vi "Experiment 24.vi"() -> ()   [LabVIEW 2026]
doc: "Experiment 24\nThis experiment (24) is like experiment 23 but uses 11 loops instead of 10."
uses:
  <vilib>/AdvancedString/1D String Array to Delimited String (string).vi
  <vilib>/Analysis/baseanly.llb/Mean (DBL).vi
  <vilib>/Analysis/NI_AALBase.lvlib
panel:
  out "No. Of Iterations Executed - Loop 11":i32
  out "Output - Loop 11":dbl[](array[numeric]) format="%.3f"
  out "No. Of Iterations As Block Of Text (easy to copy into Excel)":string
  out "No. Of Iterations Executed - Loop 10":i32
  out "Output - Loop 10":dbl[](array[numeric]) format="%.3f"
  out "No. Of Iterations Executed - Loop 9":i32
  out "Output - Loop 9":dbl[](array[numeric]) format="%.3f"
  out "No. Of Iterations Executed - Loop 8":i32
  out "Output - Loop 8":dbl[](array[numeric]) format="%.3f"
  out "No. Of Iterations Executed - Loop 7":i32
  out "Output - Loop 7":dbl[](array[numeric]) format="%.3f"
  out "No. Of Iterations Executed - Loop 6":i32
  out "Output - Loop 6":dbl[](array[numeric]) format="%.3f"
  out "No. Of Iterations Executed - Loop 5":i32
  out "Output - Loop 5":dbl[](array[numeric]) format="%.3f"
  out "No. Of Iterations Executed - Loop 4":i32
  out "Output - Loop 4":dbl[](array[numeric]) format="%.3f"
  out "No. Of Iterations Executed - Loop 3":i32
  out "Output - Loop 3":dbl[](array[numeric]) format="%.3f"
  out "Avg. No. Of Iterations Executed - All Loops":dbl format="%.1f"
  out "No. Of Iterations Executed - Loop 2":i32
  out "Output - Loop 2":dbl[](array[numeric]) format="%.3f"
  out "No. Of Iterations Executed - Loop 1":i32
  out "Output - Loop 1":dbl[](array[numeric]) format="%.3f"
  out "Stop VI?":bool
  # "Experiment 24"
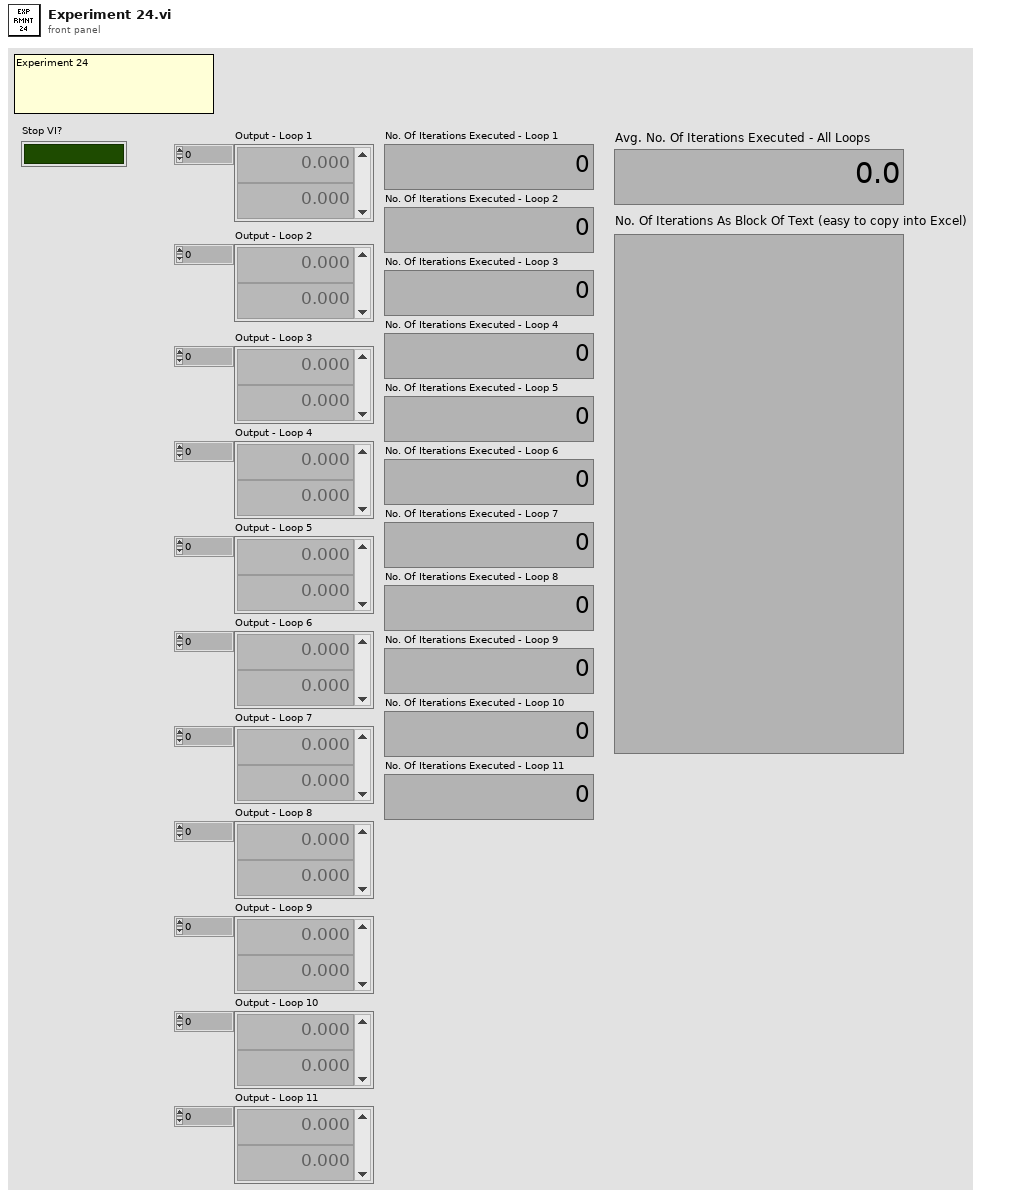
[diagram p1: front panel]
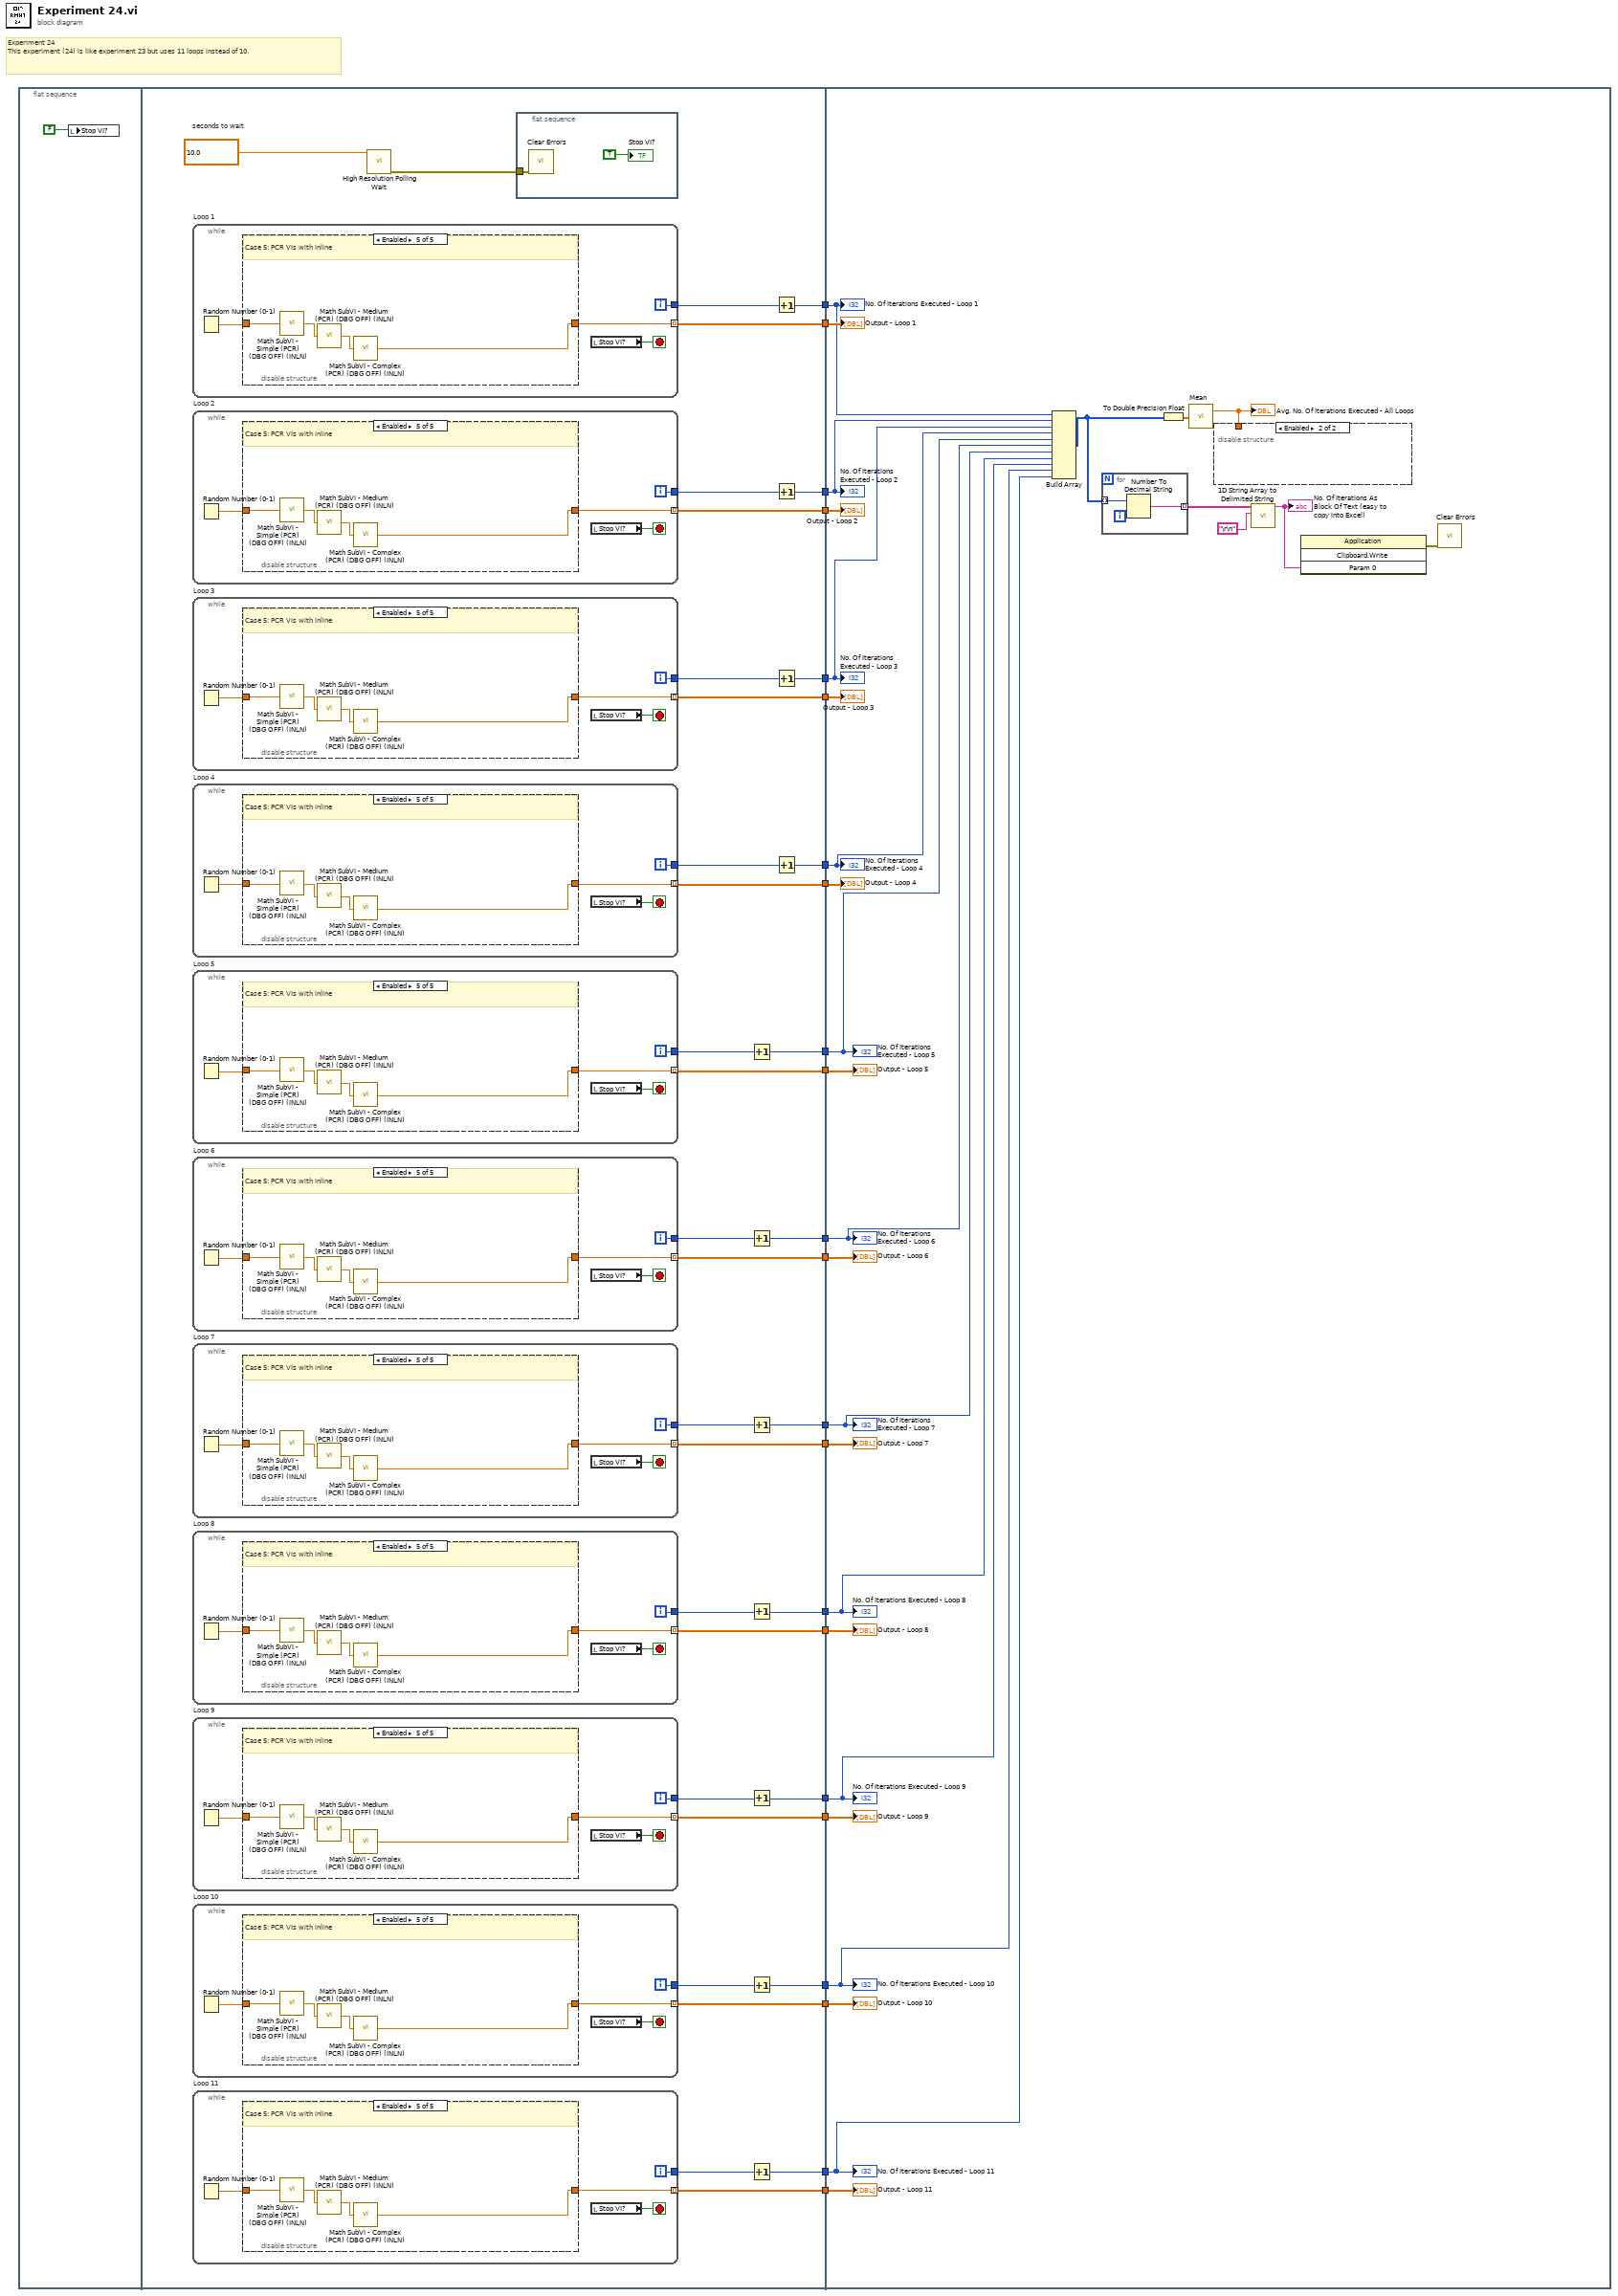
[diagram p0: block diagram]
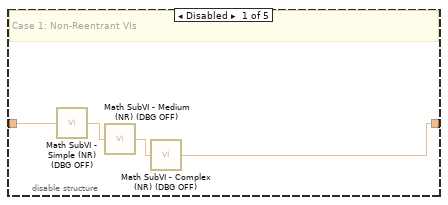
[diagram p2: hidden frame]
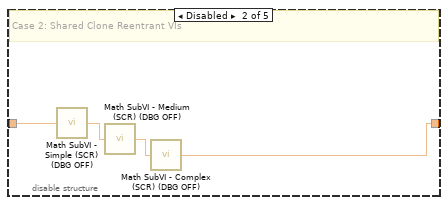
[diagram p3: hidden frame]
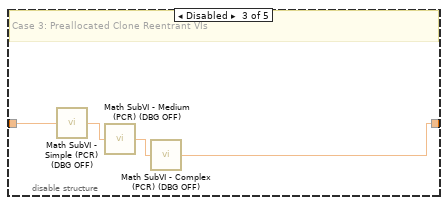
[diagram p4: hidden frame]
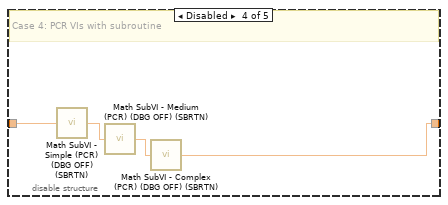
[diagram p5: hidden frame]
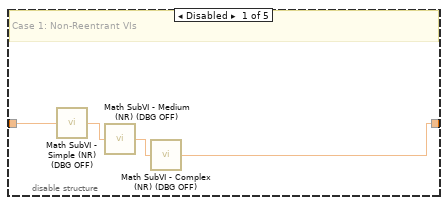
[diagram p6: hidden frame]
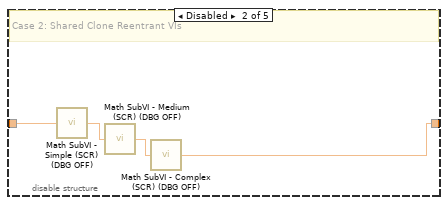
[diagram p7: hidden frame]
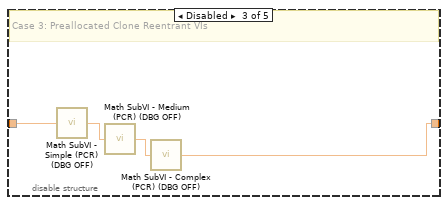
[diagram p8: hidden frame]
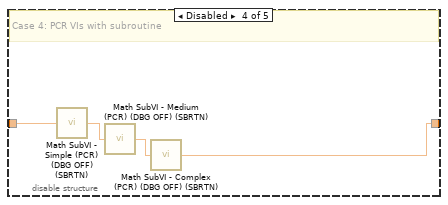
[diagram p9: hidden frame]
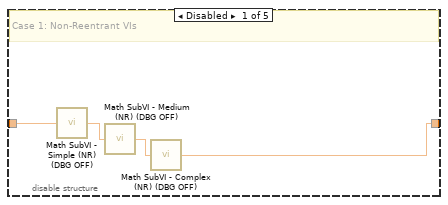
[diagram p10: hidden frame]
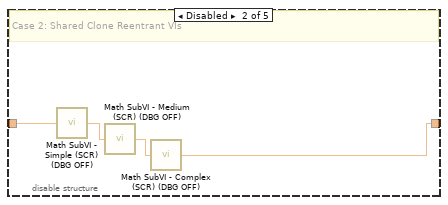
[diagram p11: hidden frame]
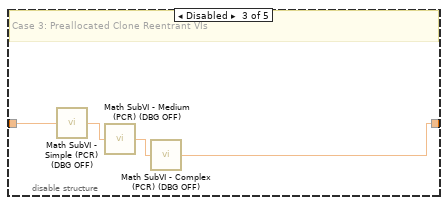
[diagram p12: hidden frame]
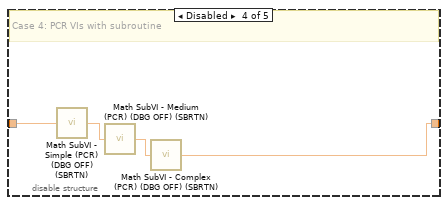
[diagram p13: hidden frame]
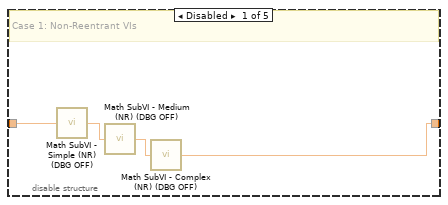
[diagram p14: hidden frame]
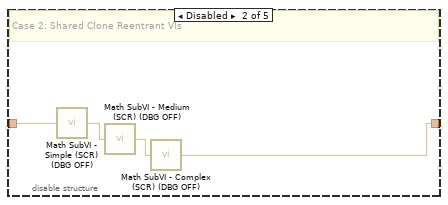
[diagram p15: hidden frame]
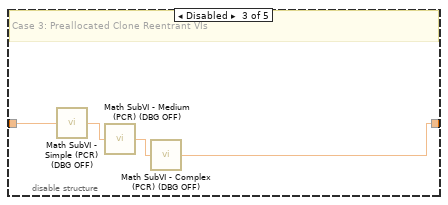
[diagram p16: hidden frame]
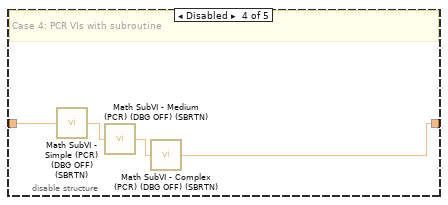
[diagram p17: hidden frame]
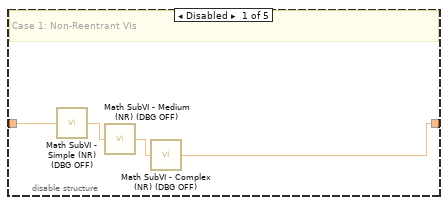
[diagram p18: hidden frame]
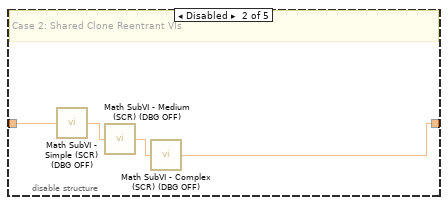
[diagram p19: hidden frame]
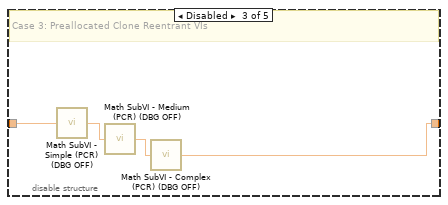
[diagram p20: hidden frame]
diagram:
  # "Experiment 24\nThis experiment (24) is like experiment 23 but uses 11 loops instead of 10."
  n1 = flat-sequence {
    tunnel: [w56] -> w22
    tunnel: [w54] -> w21
    tunnel: [w53] -> w20
    tunnel: [w44] -> w19
    tunnel: [w52] -> w18
    tunnel: [w42] -> w17
    tunnel: [w40] -> w16
    tunnel: [w51] -> w15
    tunnel: [w38] -> w14
    tunnel: [w50] -> w13
    tunnel: [w36] -> w12
    tunnel: [w45] -> w11
    tunnel: [w34] -> w10
    tunnel: [w46] -> w9
    tunnel: [w32] -> w8
    tunnel: [w47] -> w7
    tunnel: [w30] -> w6
    tunnel: [w48] -> w5
    tunnel: [w27] -> w4
    tunnel: [w49] -> w3
    tunnel: [w26] -> w2
    tunnel: [w24] -> w1
    tunnel: w22 -> [w353]
    tunnel: w21 -> [w351]
    tunnel: w20 -> [w350]
    tunnel: w19 -> [w352]
    tunnel: w18 -> [w346]
    tunnel: w17 -> [w348]
    tunnel: w16 -> [w347]
    tunnel: w15 -> [w345]
    tunnel: w14 -> [w343]
    tunnel: w13 -> [w337]
    tunnel: w12 -> [w342]
    tunnel: w11 -> [w336]
    tunnel: w10 -> [w341]
    tunnel: w9 -> [w335]
    tunnel: w8 -> [w340]
    tunnel: w7 -> [w334]
    tunnel: w6 -> [w339]
    tunnel: w5 -> [w333]
    tunnel: w4 -> [w338]
    tunnel: w3 -> [w332]
    tunnel: w2 -> [w326]
    tunnel: w1 -> [w325]
    frame #0 {
      n2 = local write "Stop VI?"(FALSE) -> ()
    }
    frame #1 {
      w58 = 10.0  # seconds to wait
      n3 = while "Loop 1" {
        tunnel: [w300] -> w56 mode=indexing
        tunnel: [w301] -> w55
        i -> [w301]
        stop <- w302 stop-if-true
        n4 = Random Number (0-1)() -> (number: 0 to 1=w299:dbl)
        n5 = disable-structure shown="Enabled" {
          disable-tunnel: w299 -> [w306 w310 w314 w318 w322]
          disable-tunnel: [w305 w309 w313 w317 w321] -> w300
          frame Disabled {
            # "Case 1: Non-Reentrant VIs"
            n6 = call "Math SubVI - Simple (NR) (DBG OFF).vi"("Input"=w306) -> ("Output"=w303:dbl)
            n7 = call "Math SubVI - Medium (NR) (DBG OFF).vi"("Input"=w303) -> ("Output"=w304:dbl)
            n8 = call "Math SubVI - Complex (NR) (DBG OFF).vi"("Input"=w304) -> ("Output"=w305:dbl)
          }
          frame Disabled {
            # "Case 2: Shared Clone Reentrant VIs"
            n9 = call "Math SubVI - Simple (SCR) (DBG OFF).vi"("Input"=w310) -> ("Output"=w307:dbl)
            n10 = call "Math SubVI - Medium (SCR) (DBG OFF).vi"("Input"=w307) -> ("Output"=w308:dbl)
            n11 = call "Math SubVI - Complex (SCR) (DBG OFF).vi"("Input"=w308) -> ("Output"=w309:dbl)
          }
          frame Disabled {
            # "Case 3: Preallocated Clone Reentrant VIs"
            n12 = call "Math SubVI - Simple (PCR) (DBG OFF).vi"("Input"=w314) -> ("Output"=w311:dbl)
            n13 = call "Math SubVI - Medium (PCR) (DBG OFF).vi"("Input"=w311) -> ("Output"=w312:dbl)
            n14 = call "Math SubVI - Complex (PCR) (DBG OFF).vi"("Input"=w312) -> ("Output"=w313:dbl)
          }
          frame Disabled {
            # "Case 4: PCR VIs with subroutine"
            n15 = call "Math SubVI - Simple (PCR) (DBG OFF) (SBRTN).vi"("Input"=w318) -> ("Output"=w315:dbl)
            n16 = call "Math SubVI - Medium (PCR) (DBG OFF) (SBRTN).vi"("Input"=w315) -> ("Output"=w316:dbl)
            n17 = call "Math SubVI - Complex (PCR) (DBG OFF) (SBRTN).vi"("Input"=w316) -> ("Output"=w317:dbl)
          }
          frame Enabled {
            # "Case 5: PCR VIs with inline"
            n18 = call "Math SubVI - Simple (PCR) (DBG OFF) (INLN).vi"("Input"=w322) -> ("Output"=w319:dbl)
            n19 = call "Math SubVI - Medium (PCR) (DBG OFF) (INLN).vi"("Input"=w319) -> ("Output"=w320:dbl)
            n20 = call "Math SubVI - Complex (PCR) (DBG OFF) (INLN).vi"("Input"=w320) -> ("Output"=w321:dbl)
          }
        }
        n21 = local read "Stop VI?"() -> (w302:bool)
      }
      n22 = while "Loop 2" {
        tunnel: [w276] -> w44 mode=indexing
        tunnel: [w277] -> w43
        i -> [w277]
        stop <- w278 stop-if-true
        n23 = Random Number (0-1)() -> (number: 0 to 1=w275:dbl)
        n24 = disable-structure shown="Enabled" {
          disable-tunnel: w275 -> [w282 w286 w290 w294 w298]
          disable-tunnel: [w281 w285 w289 w293 w297] -> w276
          frame Disabled {
            # "Case 1: Non-Reentrant VIs"
            n25 = call "Math SubVI - Simple (NR) (DBG OFF).vi"("Input"=w282) -> ("Output"=w279:dbl)
            n26 = call "Math SubVI - Medium (NR) (DBG OFF).vi"("Input"=w279) -> ("Output"=w280:dbl)
            n27 = call "Math SubVI - Complex (NR) (DBG OFF).vi"("Input"=w280) -> ("Output"=w281:dbl)
          }
          frame Disabled {
            # "Case 2: Shared Clone Reentrant VIs"
            n28 = call "Math SubVI - Simple (SCR) (DBG OFF).vi"("Input"=w286) -> ("Output"=w283:dbl)
            n29 = call "Math SubVI - Medium (SCR) (DBG OFF).vi"("Input"=w283) -> ("Output"=w284:dbl)
            n30 = call "Math SubVI - Complex (SCR) (DBG OFF).vi"("Input"=w284) -> ("Output"=w285:dbl)
          }
          frame Disabled {
            # "Case 3: Preallocated Clone Reentrant VIs"
            n31 = call "Math SubVI - Simple (PCR) (DBG OFF).vi"("Input"=w290) -> ("Output"=w287:dbl)
            n32 = call "Math SubVI - Medium (PCR) (DBG OFF).vi"("Input"=w287) -> ("Output"=w288:dbl)
            n33 = call "Math SubVI - Complex (PCR) (DBG OFF).vi"("Input"=w288) -> ("Output"=w289:dbl)
          }
          frame Disabled {
            # "Case 4: PCR VIs with subroutine"
            n34 = call "Math SubVI - Simple (PCR) (DBG OFF) (SBRTN).vi"("Input"=w294) -> ("Output"=w291:dbl)
            n35 = call "Math SubVI - Medium (PCR) (DBG OFF) (SBRTN).vi"("Input"=w291) -> ("Output"=w292:dbl)
            n36 = call "Math SubVI - Complex (PCR) (DBG OFF) (SBRTN).vi"("Input"=w292) -> ("Output"=w293:dbl)
          }
          frame Enabled {
            # "Case 5: PCR VIs with inline"
            n37 = call "Math SubVI - Simple (PCR) (DBG OFF) (INLN).vi"("Input"=w298) -> ("Output"=w295:dbl)
            n38 = call "Math SubVI - Medium (PCR) (DBG OFF) (INLN).vi"("Input"=w295) -> ("Output"=w296:dbl)
            n39 = call "Math SubVI - Complex (PCR) (DBG OFF) (INLN).vi"("Input"=w296) -> ("Output"=w297:dbl)
          }
        }
        n40 = local read "Stop VI?"() -> (w278:bool)
      }
      n41 = while "Loop 3" {
        tunnel: [w252] -> w42 mode=indexing
        tunnel: [w253] -> w41
        i -> [w253]
        stop <- w254 stop-if-true
        n42 = Random Number (0-1)() -> (number: 0 to 1=w251:dbl)
        n43 = disable-structure shown="Enabled" {
          disable-tunnel: w251 -> [w258 w262 w266 w270 w274]
          disable-tunnel: [w257 w261 w265 w269 w273] -> w252
          frame Disabled {
            # "Case 1: Non-Reentrant VIs"
            n44 = call "Math SubVI - Simple (NR) (DBG OFF).vi"("Input"=w258) -> ("Output"=w255:dbl)
            n45 = call "Math SubVI - Medium (NR) (DBG OFF).vi"("Input"=w255) -> ("Output"=w256:dbl)
            n46 = call "Math SubVI - Complex (NR) (DBG OFF).vi"("Input"=w256) -> ("Output"=w257:dbl)
          }
          frame Disabled {
            # "Case 2: Shared Clone Reentrant VIs"
            n47 = call "Math SubVI - Simple (SCR) (DBG OFF).vi"("Input"=w262) -> ("Output"=w259:dbl)
            n48 = call "Math SubVI - Medium (SCR) (DBG OFF).vi"("Input"=w259) -> ("Output"=w260:dbl)
            n49 = call "Math SubVI - Complex (SCR) (DBG OFF).vi"("Input"=w260) -> ("Output"=w261:dbl)
          }
          frame Disabled {
            # "Case 3: Preallocated Clone Reentrant VIs"
            n50 = call "Math SubVI - Simple (PCR) (DBG OFF).vi"("Input"=w266) -> ("Output"=w263:dbl)
            n51 = call "Math SubVI - Medium (PCR) (DBG OFF).vi"("Input"=w263) -> ("Output"=w264:dbl)
            n52 = call "Math SubVI - Complex (PCR) (DBG OFF).vi"("Input"=w264) -> ("Output"=w265:dbl)
          }
          frame Disabled {
            # "Case 4: PCR VIs with subroutine"
            n53 = call "Math SubVI - Simple (PCR) (DBG OFF) (SBRTN).vi"("Input"=w270) -> ("Output"=w267:dbl)
            n54 = call "Math SubVI - Medium (PCR) (DBG OFF) (SBRTN).vi"("Input"=w267) -> ("Output"=w268:dbl)
            n55 = call "Math SubVI - Complex (PCR) (DBG OFF) (SBRTN).vi"("Input"=w268) -> ("Output"=w269:dbl)
          }
          frame Enabled {
            # "Case 5: PCR VIs with inline"
            n56 = call "Math SubVI - Simple (PCR) (DBG OFF) (INLN).vi"("Input"=w274) -> ("Output"=w271:dbl)
            n57 = call "Math SubVI - Medium (PCR) (DBG OFF) (INLN).vi"("Input"=w271) -> ("Output"=w272:dbl)
            n58 = call "Math SubVI - Complex (PCR) (DBG OFF) (INLN).vi"("Input"=w272) -> ("Output"=w273:dbl)
          }
        }
        n59 = local read "Stop VI?"() -> (w254:bool)
      }
      n60 = while "Loop 4" {
        tunnel: [w228] -> w40 mode=indexing
        tunnel: [w229] -> w39
        i -> [w229]
        stop <- w230 stop-if-true
        n61 = Random Number (0-1)() -> (number: 0 to 1=w227:dbl)
        n62 = disable-structure shown="Enabled" {
          disable-tunnel: w227 -> [w234 w238 w242 w246 w250]
          disable-tunnel: [w233 w237 w241 w245 w249] -> w228
          frame Disabled {
            # "Case 1: Non-Reentrant VIs"
            n63 = call "Math SubVI - Simple (NR) (DBG OFF).vi"("Input"=w234) -> ("Output"=w231:dbl)
            n64 = call "Math SubVI - Medium (NR) (DBG OFF).vi"("Input"=w231) -> ("Output"=w232:dbl)
            n65 = call "Math SubVI - Complex (NR) (DBG OFF).vi"("Input"=w232) -> ("Output"=w233:dbl)
          }
          frame Disabled {
            # "Case 2: Shared Clone Reentrant VIs"
            n66 = call "Math SubVI - Simple (SCR) (DBG OFF).vi"("Input"=w238) -> ("Output"=w235:dbl)
            n67 = call "Math SubVI - Medium (SCR) (DBG OFF).vi"("Input"=w235) -> ("Output"=w236:dbl)
            n68 = call "Math SubVI - Complex (SCR) (DBG OFF).vi"("Input"=w236) -> ("Output"=w237:dbl)
          }
          frame Disabled {
            # "Case 3: Preallocated Clone Reentrant VIs"
            n69 = call "Math SubVI - Simple (PCR) (DBG OFF).vi"("Input"=w242) -> ("Output"=w239:dbl)
            n70 = call "Math SubVI - Medium (PCR) (DBG OFF).vi"("Input"=w239) -> ("Output"=w240:dbl)
            n71 = call "Math SubVI - Complex (PCR) (DBG OFF).vi"("Input"=w240) -> ("Output"=w241:dbl)
          }
          frame Disabled {
            # "Case 4: PCR VIs with subroutine"
            n72 = call "Math SubVI - Simple (PCR) (DBG OFF) (SBRTN).vi"("Input"=w246) -> ("Output"=w243:dbl)
            n73 = call "Math SubVI - Medium (PCR) (DBG OFF) (SBRTN).vi"("Input"=w243) -> ("Output"=w244:dbl)
            n74 = call "Math SubVI - Complex (PCR) (DBG OFF) (SBRTN).vi"("Input"=w244) -> ("Output"=w245:dbl)
          }
          frame Enabled {
            # "Case 5: PCR VIs with inline"
            n75 = call "Math SubVI - Simple (PCR) (DBG OFF) (INLN).vi"("Input"=w250) -> ("Output"=w247:dbl)
            n76 = call "Math SubVI - Medium (PCR) (DBG OFF) (INLN).vi"("Input"=w247) -> ("Output"=w248:dbl)
            n77 = call "Math SubVI - Complex (PCR) (DBG OFF) (INLN).vi"("Input"=w248) -> ("Output"=w249:dbl)
          }
        }
        n78 = local read "Stop VI?"() -> (w230:bool)
      }
      n79 = while "Loop 5" {
        tunnel: [w204] -> w38 mode=indexing
        tunnel: [w205] -> w37
        i -> [w205]
        stop <- w206 stop-if-true
        n80 = Random Number (0-1)() -> (number: 0 to 1=w203:dbl)
        n81 = disable-structure shown="Enabled" {
          disable-tunnel: w203 -> [w210 w214 w218 w222 w226]
          disable-tunnel: [w209 w213 w217 w221 w225] -> w204
          frame Disabled {
            # "Case 1: Non-Reentrant VIs"
            n82 = call "Math SubVI - Simple (NR) (DBG OFF).vi"("Input"=w210) -> ("Output"=w207:dbl)
            n83 = call "Math SubVI - Medium (NR) (DBG OFF).vi"("Input"=w207) -> ("Output"=w208:dbl)
            n84 = call "Math SubVI - Complex (NR) (DBG OFF).vi"("Input"=w208) -> ("Output"=w209:dbl)
          }
          frame Disabled {
            # "Case 2: Shared Clone Reentrant VIs"
            n85 = call "Math SubVI - Simple (SCR) (DBG OFF).vi"("Input"=w214) -> ("Output"=w211:dbl)
            n86 = call "Math SubVI - Medium (SCR) (DBG OFF).vi"("Input"=w211) -> ("Output"=w212:dbl)
            n87 = call "Math SubVI - Complex (SCR) (DBG OFF).vi"("Input"=w212) -> ("Output"=w213:dbl)
          }
          frame Disabled {
            # "Case 3: Preallocated Clone Reentrant VIs"
            n88 = call "Math SubVI - Simple (PCR) (DBG OFF).vi"("Input"=w218) -> ("Output"=w215:dbl)
            n89 = call "Math SubVI - Medium (PCR) (DBG OFF).vi"("Input"=w215) -> ("Output"=w216:dbl)
            n90 = call "Math SubVI - Complex (PCR) (DBG OFF).vi"("Input"=w216) -> ("Output"=w217:dbl)
          }
          frame Disabled {
            # "Case 4: PCR VIs with subroutine"
            n91 = call "Math SubVI - Simple (PCR) (DBG OFF) (SBRTN).vi"("Input"=w222) -> ("Output"=w219:dbl)
            n92 = call "Math SubVI - Medium (PCR) (DBG OFF) (SBRTN).vi"("Input"=w219) -> ("Output"=w220:dbl)
            n93 = call "Math SubVI - Complex (PCR) (DBG OFF) (SBRTN).vi"("Input"=w220) -> ("Output"=w221:dbl)
          }
          frame Enabled {
            # "Case 5: PCR VIs with inline"
            n94 = call "Math SubVI - Simple (PCR) (DBG OFF) (INLN).vi"("Input"=w226) -> ("Output"=w223:dbl)
            n95 = call "Math SubVI - Medium (PCR) (DBG OFF) (INLN).vi"("Input"=w223) -> ("Output"=w224:dbl)
            n96 = call "Math SubVI - Complex (PCR) (DBG OFF) (INLN).vi"("Input"=w224) -> ("Output"=w225:dbl)
          }
        }
        n97 = local read "Stop VI?"() -> (w206:bool)
      }
      n98 = while "Loop 6" {
        tunnel: [w180] -> w36 mode=indexing
        tunnel: [w181] -> w35
        i -> [w181]
        stop <- w182 stop-if-true
        n99 = Random Number (0-1)() -> (number: 0 to 1=w179:dbl)
        n100 = disable-structure shown="Enabled" {
          disable-tunnel: w179 -> [w186 w190 w194 w198 w202]
          disable-tunnel: [w185 w189 w193 w197 w201] -> w180
          frame Disabled {
            # "Case 1: Non-Reentrant VIs"
            n101 = call "Math SubVI - Simple (NR) (DBG OFF).vi"("Input"=w186) -> ("Output"=w183:dbl)
            n102 = call "Math SubVI - Medium (NR) (DBG OFF).vi"("Input"=w183) -> ("Output"=w184:dbl)
            n103 = call "Math SubVI - Complex (NR) (DBG OFF).vi"("Input"=w184) -> ("Output"=w185:dbl)
          }
          frame Disabled {
            # "Case 2: Shared Clone Reentrant VIs"
            n104 = call "Math SubVI - Simple (SCR) (DBG OFF).vi"("Input"=w190) -> ("Output"=w187:dbl)
            n105 = call "Math SubVI - Medium (SCR) (DBG OFF).vi"("Input"=w187) -> ("Output"=w188:dbl)
            n106 = call "Math SubVI - Complex (SCR) (DBG OFF).vi"("Input"=w188) -> ("Output"=w189:dbl)
          }
          frame Disabled {
            # "Case 3: Preallocated Clone Reentrant VIs"
            n107 = call "Math SubVI - Simple (PCR) (DBG OFF).vi"("Input"=w194) -> ("Output"=w191:dbl)
            n108 = call "Math SubVI - Medium (PCR) (DBG OFF).vi"("Input"=w191) -> ("Output"=w192:dbl)
            n109 = call "Math SubVI - Complex (PCR) (DBG OFF).vi"("Input"=w192) -> ("Output"=w193:dbl)
          }
          frame Disabled {
            # "Case 4: PCR VIs with subroutine"
            n110 = call "Math SubVI - Simple (PCR) (DBG OFF) (SBRTN).vi"("Input"=w198) -> ("Output"=w195:dbl)
            n111 = call "Math SubVI - Medium (PCR) (DBG OFF) (SBRTN).vi"("Input"=w195) -> ("Output"=w196:dbl)
            n112 = call "Math SubVI - Complex (PCR) (DBG OFF) (SBRTN).vi"("Input"=w196) -> ("Output"=w197:dbl)
          }
          frame Enabled {
            # "Case 5: PCR VIs with inline"
            n113 = call "Math SubVI - Simple (PCR) (DBG OFF) (INLN).vi"("Input"=w202) -> ("Output"=w199:dbl)
            n114 = call "Math SubVI - Medium (PCR) (DBG OFF) (INLN).vi"("Input"=w199) -> ("Output"=w200:dbl)
            n115 = call "Math SubVI - Complex (PCR) (DBG OFF) (INLN).vi"("Input"=w200) -> ("Output"=w201:dbl)
          }
        }
        n116 = local read "Stop VI?"() -> (w182:bool)
      }
      n117 = while "Loop 7" {
        tunnel: [w156] -> w34 mode=indexing
        tunnel: [w157] -> w33
        i -> [w157]
        stop <- w158 stop-if-true
        n118 = Random Number (0-1)() -> (number: 0 to 1=w155:dbl)
        n119 = disable-structure shown="Enabled" {
          disable-tunnel: w155 -> [w162 w166 w170 w174 w178]
          disable-tunnel: [w161 w165 w169 w173 w177] -> w156
          frame Disabled {
            # "Case 1: Non-Reentrant VIs"
            n120 = call "Math SubVI - Simple (NR) (DBG OFF).vi"("Input"=w162) -> ("Output"=w159:dbl)
            n121 = call "Math SubVI - Medium (NR) (DBG OFF).vi"("Input"=w159) -> ("Output"=w160:dbl)
            n122 = call "Math SubVI - Complex (NR) (DBG OFF).vi"("Input"=w160) -> ("Output"=w161:dbl)
          }
          frame Disabled {
            # "Case 2: Shared Clone Reentrant VIs"
            n123 = call "Math SubVI - Simple (SCR) (DBG OFF).vi"("Input"=w166) -> ("Output"=w163:dbl)
            n124 = call "Math SubVI - Medium (SCR) (DBG OFF).vi"("Input"=w163) -> ("Output"=w164:dbl)
            n125 = call "Math SubVI - Complex (SCR) (DBG OFF).vi"("Input"=w164) -> ("Output"=w165:dbl)
          }
          frame Disabled {
            # "Case 3: Preallocated Clone Reentrant VIs"
            n126 = call "Math SubVI - Simple (PCR) (DBG OFF).vi"("Input"=w170) -> ("Output"=w167:dbl)
            n127 = call "Math SubVI - Medium (PCR) (DBG OFF).vi"("Input"=w167) -> ("Output"=w168:dbl)
            n128 = call "Math SubVI - Complex (PCR) (DBG OFF).vi"("Input"=w168) -> ("Output"=w169:dbl)
          }
          frame Disabled {
            # "Case 4: PCR VIs with subroutine"
            n129 = call "Math SubVI - Simple (PCR) (DBG OFF) (SBRTN).vi"("Input"=w174) -> ("Output"=w171:dbl)
            n130 = call "Math SubVI - Medium (PCR) (DBG OFF) (SBRTN).vi"("Input"=w171) -> ("Output"=w172:dbl)
            n131 = call "Math SubVI - Complex (PCR) (DBG OFF) (SBRTN).vi"("Input"=w172) -> ("Output"=w173:dbl)
          }
          frame Enabled {
            # "Case 5: PCR VIs with inline"
            n132 = call "Math SubVI - Simple (PCR) (DBG OFF) (INLN).vi"("Input"=w178) -> ("Output"=w175:dbl)
            n133 = call "Math SubVI - Medium (PCR) (DBG OFF) (INLN).vi"("Input"=w175) -> ("Output"=w176:dbl)
            n134 = call "Math SubVI - Complex (PCR) (DBG OFF) (INLN).vi"("Input"=w176) -> ("Output"=w177:dbl)
          }
        }
        n135 = local read "Stop VI?"() -> (w158:bool)
      }
      n136 = while "Loop 8" {
        tunnel: [w132] -> w32 mode=indexing
        tunnel: [w133] -> w31
        i -> [w133]
        stop <- w134 stop-if-true
        n137 = Random Number (0-1)() -> (number: 0 to 1=w131:dbl)
        n138 = disable-structure shown="Enabled" {
          disable-tunnel: w131 -> [w138 w142 w146 w150 w154]
          disable-tunnel: [w137 w141 w145 w149 w153] -> w132
          frame Disabled {
            # "Case 1: Non-Reentrant VIs"
            n139 = call "Math SubVI - Simple (NR) (DBG OFF).vi"("Input"=w138) -> ("Output"=w135:dbl)
            n140 = call "Math SubVI - Medium (NR) (DBG OFF).vi"("Input"=w135) -> ("Output"=w136:dbl)
            n141 = call "Math SubVI - Complex (NR) (DBG OFF).vi"("Input"=w136) -> ("Output"=w137:dbl)
          }
          frame Disabled {
            # "Case 2: Shared Clone Reentrant VIs"
            n142 = call "Math SubVI - Simple (SCR) (DBG OFF).vi"("Input"=w142) -> ("Output"=w139:dbl)
            n143 = call "Math SubVI - Medium (SCR) (DBG OFF).vi"("Input"=w139) -> ("Output"=w140:dbl)
            n144 = call "Math SubVI - Complex (SCR) (DBG OFF).vi"("Input"=w140) -> ("Output"=w141:dbl)
          }
          frame Disabled {
            # "Case 3: Preallocated Clone Reentrant VIs"
            n145 = call "Math SubVI - Simple (PCR) (DBG OFF).vi"("Input"=w146) -> ("Output"=w143:dbl)
            n146 = call "Math SubVI - Medium (PCR) (DBG OFF).vi"("Input"=w143) -> ("Output"=w144:dbl)
            n147 = call "Math SubVI - Complex (PCR) (DBG OFF).vi"("Input"=w144) -> ("Output"=w145:dbl)
          }
          frame Disabled {
            # "Case 4: PCR VIs with subroutine"
            n148 = call "Math SubVI - Simple (PCR) (DBG OFF) (SBRTN).vi"("Input"=w150) -> ("Output"=w147:dbl)
            n149 = call "Math SubVI - Medium (PCR) (DBG OFF) (SBRTN).vi"("Input"=w147) -> ("Output"=w148:dbl)
            n150 = call "Math SubVI - Complex (PCR) (DBG OFF) (SBRTN).vi"("Input"=w148) -> ("Output"=w149:dbl)
          }
          frame Enabled {
            # "Case 5: PCR VIs with inline"
            n151 = call "Math SubVI - Simple (PCR) (DBG OFF) (INLN).vi"("Input"=w154) -> ("Output"=w151:dbl)
            n152 = call "Math SubVI - Medium (PCR) (DBG OFF) (INLN).vi"("Input"=w151) -> ("Output"=w152:dbl)
            n153 = call "Math SubVI - Complex (PCR) (DBG OFF) (INLN).vi"("Input"=w152) -> ("Output"=w153:dbl)
          }
        }
        n154 = local read "Stop VI?"() -> (w134:bool)
      }
      n155 = while "Loop 9" {
        tunnel: [w108] -> w30 mode=indexing
        tunnel: [w109] -> w29
        i -> [w109]
        stop <- w110 stop-if-true
        n156 = Random Number (0-1)() -> (number: 0 to 1=w107:dbl)
        n157 = disable-structure shown="Enabled" {
          disable-tunnel: w107 -> [w114 w118 w122 w126 w130]
          disable-tunnel: [w113 w117 w121 w125 w129] -> w108
          frame Disabled {
            # "Case 1: Non-Reentrant VIs"
            n158 = call "Math SubVI - Simple (NR) (DBG OFF).vi"("Input"=w114) -> ("Output"=w111:dbl)
            n159 = call "Math SubVI - Medium (NR) (DBG OFF).vi"("Input"=w111) -> ("Output"=w112:dbl)
            n160 = call "Math SubVI - Complex (NR) (DBG OFF).vi"("Input"=w112) -> ("Output"=w113:dbl)
          }
          frame Disabled {
            # "Case 2: Shared Clone Reentrant VIs"
            n161 = call "Math SubVI - Simple (SCR) (DBG OFF).vi"("Input"=w118) -> ("Output"=w115:dbl)
            n162 = call "Math SubVI - Medium (SCR) (DBG OFF).vi"("Input"=w115) -> ("Output"=w116:dbl)
            n163 = call "Math SubVI - Complex (SCR) (DBG OFF).vi"("Input"=w116) -> ("Output"=w117:dbl)
          }
          frame Disabled {
            # "Case 3: Preallocated Clone Reentrant VIs"
            n164 = call "Math SubVI - Simple (PCR) (DBG OFF).vi"("Input"=w122) -> ("Output"=w119:dbl)
            n165 = call "Math SubVI - Medium (PCR) (DBG OFF).vi"("Input"=w119) -> ("Output"=w120:dbl)
            n166 = call "Math SubVI - Complex (PCR) (DBG OFF).vi"("Input"=w120) -> ("Output"=w121:dbl)
          }
          frame Disabled {
            # "Case 4: PCR VIs with subroutine"
            n167 = call "Math SubVI - Simple (PCR) (DBG OFF) (SBRTN).vi"("Input"=w126) -> ("Output"=w123:dbl)
            n168 = call "Math SubVI - Medium (PCR) (DBG OFF) (SBRTN).vi"("Input"=w123) -> ("Output"=w124:dbl)
            n169 = call "Math SubVI - Complex (PCR) (DBG OFF) (SBRTN).vi"("Input"=w124) -> ("Output"=w125:dbl)
          }
          frame Enabled {
            # "Case 5: PCR VIs with inline"
            n170 = call "Math SubVI - Simple (PCR) (DBG OFF) (INLN).vi"("Input"=w130) -> ("Output"=w127:dbl)
            n171 = call "Math SubVI - Medium (PCR) (DBG OFF) (INLN).vi"("Input"=w127) -> ("Output"=w128:dbl)
            n172 = call "Math SubVI - Complex (PCR) (DBG OFF) (INLN).vi"("Input"=w128) -> ("Output"=w129:dbl)
          }
        }
        n173 = local read "Stop VI?"() -> (w110:bool)
      }
      n174 = while "Loop 10" {
        tunnel: [w84] -> w27 mode=indexing
        tunnel: [w85] -> w28
        i -> [w85]
        stop <- w86 stop-if-true
        n175 = Random Number (0-1)() -> (number: 0 to 1=w83:dbl)
        n176 = disable-structure shown="Enabled" {
          disable-tunnel: w83 -> [w90 w94 w98 w102 w106]
          disable-tunnel: [w89 w93 w97 w101 w105] -> w84
          frame Disabled {
            # "Case 1: Non-Reentrant VIs"
            n177 = call "Math SubVI - Simple (NR) (DBG OFF).vi"("Input"=w90) -> ("Output"=w87:dbl)
            n178 = call "Math SubVI - Medium (NR) (DBG OFF).vi"("Input"=w87) -> ("Output"=w88:dbl)
            n179 = call "Math SubVI - Complex (NR) (DBG OFF).vi"("Input"=w88) -> ("Output"=w89:dbl)
          }
          frame Disabled {
            # "Case 2: Shared Clone Reentrant VIs"
            n180 = call "Math SubVI - Simple (SCR) (DBG OFF).vi"("Input"=w94) -> ("Output"=w91:dbl)
            n181 = call "Math SubVI - Medium (SCR) (DBG OFF).vi"("Input"=w91) -> ("Output"=w92:dbl)
            n182 = call "Math SubVI - Complex (SCR) (DBG OFF).vi"("Input"=w92) -> ("Output"=w93:dbl)
          }
          frame Disabled {
            # "Case 3: Preallocated Clone Reentrant VIs"
            n183 = call "Math SubVI - Simple (PCR) (DBG OFF).vi"("Input"=w98) -> ("Output"=w95:dbl)
            n184 = call "Math SubVI - Medium (PCR) (DBG OFF).vi"("Input"=w95) -> ("Output"=w96:dbl)
            n185 = call "Math SubVI - Complex (PCR) (DBG OFF).vi"("Input"=w96) -> ("Output"=w97:dbl)
          }
          frame Disabled {
            # "Case 4: PCR VIs with subroutine"
            n186 = call "Math SubVI - Simple (PCR) (DBG OFF) (SBRTN).vi"("Input"=w102) -> ("Output"=w99:dbl)
            n187 = call "Math SubVI - Medium (PCR) (DBG OFF) (SBRTN).vi"("Input"=w99) -> ("Output"=w100:dbl)
            n188 = call "Math SubVI - Complex (PCR) (DBG OFF) (SBRTN).vi"("Input"=w100) -> ("Output"=w101:dbl)
          }
          frame Enabled {
            # "Case 5: PCR VIs with inline"
            n189 = call "Math SubVI - Simple (PCR) (DBG OFF) (INLN).vi"("Input"=w106) -> ("Output"=w103:dbl)
            n190 = call "Math SubVI - Medium (PCR) (DBG OFF) (INLN).vi"("Input"=w103) -> ("Output"=w104:dbl)
            n191 = call "Math SubVI - Complex (PCR) (DBG OFF) (INLN).vi"("Input"=w104) -> ("Output"=w105:dbl)
          }
        }
        n192 = local read "Stop VI?"() -> (w86:bool)
      }
      n193 = while "Loop 11" {
        tunnel: [w60] -> w26 mode=indexing
        tunnel: [w61] -> w25
        i -> [w61]
        stop <- w62 stop-if-true
        n194 = Random Number (0-1)() -> (number: 0 to 1=w59:dbl)
        n195 = disable-structure shown="Enabled" {
          disable-tunnel: w59 -> [w66 w70 w74 w78 w82]
          disable-tunnel: [w65 w69 w73 w77 w81] -> w60
          frame Disabled {
            # "Case 1: Non-Reentrant VIs"
            n196 = call "Math SubVI - Simple (NR) (DBG OFF).vi"("Input"=w66) -> ("Output"=w63:dbl)
            n197 = call "Math SubVI - Medium (NR) (DBG OFF).vi"("Input"=w63) -> ("Output"=w64:dbl)
            n198 = call "Math SubVI - Complex (NR) (DBG OFF).vi"("Input"=w64) -> ("Output"=w65:dbl)
          }
          frame Disabled {
            # "Case 2: Shared Clone Reentrant VIs"
            n199 = call "Math SubVI - Simple (SCR) (DBG OFF).vi"("Input"=w70) -> ("Output"=w67:dbl)
            n200 = call "Math SubVI - Medium (SCR) (DBG OFF).vi"("Input"=w67) -> ("Output"=w68:dbl)
            n201 = call "Math SubVI - Complex (SCR) (DBG OFF).vi"("Input"=w68) -> ("Output"=w69:dbl)
          }
          frame Disabled {
            # "Case 3: Preallocated Clone Reentrant VIs"
            n202 = call "Math SubVI - Simple (PCR) (DBG OFF).vi"("Input"=w74) -> ("Output"=w71:dbl)
            n203 = call "Math SubVI - Medium (PCR) (DBG OFF).vi"("Input"=w71) -> ("Output"=w72:dbl)
            n204 = call "Math SubVI - Complex (PCR) (DBG OFF).vi"("Input"=w72) -> ("Output"=w73:dbl)
          }
          frame Disabled {
            # "Case 4: PCR VIs with subroutine"
            n205 = call "Math SubVI - Simple (PCR) (DBG OFF) (SBRTN).vi"("Input"=w78) -> ("Output"=w75:dbl)
            n206 = call "Math SubVI - Medium (PCR) (DBG OFF) (SBRTN).vi"("Input"=w75) -> ("Output"=w76:dbl)
            n207 = call "Math SubVI - Complex (PCR) (DBG OFF) (SBRTN).vi"("Input"=w76) -> ("Output"=w77:dbl)
          }
          frame Enabled {
            # "Case 5: PCR VIs with inline"
            n208 = call "Math SubVI - Simple (PCR) (DBG OFF) (INLN).vi"("Input"=w82) -> ("Output"=w79:dbl)
            n209 = call "Math SubVI - Medium (PCR) (DBG OFF) (INLN).vi"("Input"=w79) -> ("Output"=w80:dbl)
            n210 = call "Math SubVI - Complex (PCR) (DBG OFF) (INLN).vi"("Input"=w80) -> ("Output"=w81:dbl)
          }
        }
        n211 = local read "Stop VI?"() -> (w62:bool)
      }
      n212 = call <vilib>:"High Resolution Polling Wait.vi"("seconds to wait"=w58) -> ("error out"=w57:errorcluster)  [unwired: 10 in]
      n213 = flat-sequence {
        tunnel: w57 -> [w323]
        frame #0 {
          n214 = call <vilib>:"Clear Errors.vi"("error in (no error)"=w323) -> ()  [unwired: 5 in, 2 out]
          "Stop VI?" <- TRUE
        }
      }
      n215 = Increment(x=w37) -> (x+1=w50:i32)
      n216 = Increment(x=w35) -> (x+1=w45:i32)
      n217 = Increment(x=w33) -> (x+1=w46:i32)
      n218 = Increment(x=w31) -> (x+1=w47:i32)
      n219 = Increment(x=w29) -> (x+1=w48:i32)
      n220 = Increment(x=w28) -> (x+1=w49:i32)
      n221 = Increment(x=w25) -> (x+1=w24:i32)
      n222 = Increment(x=w55) -> (x+1=w54:i32)
      n223 = Increment(x=w43) -> (x+1=w53:i32)
      n224 = Increment(x=w41) -> (x+1=w52:i32)
      n225 = Increment(x=w39) -> (x+1=w51:i32)
    }
    frame #2 {
      n226 = Build Array(w351, w350, w346, w345, w337, w336, w335, w334, w333, w332, w325) -> (w331:i32[])
      n227 = for {
        tunnel: w331 -> [w357] mode=indexing
        tunnel: [w356] -> w330 mode=indexing
        n228 = Number To Decimal String(number=w357) -> (decimal integer string=w356:string)  [unwired: 1 in]
      }
      n229 = To Double Precision Float(number=w331) -> (double precision float=w344:dbl[])
      n230 = call-poly <vilib>:"Mean.vi"("X"=w344) -> ("mean"=w349:dbl)  [unwired: 1 out]
      "Avg. No. Of Iterations Executed - All Loops" <- w349
      n231 = disable-structure shown="Enabled" {
        disable-tunnel: w349 -> [w355 _]
        frame Disabled {
          n232 = call "Copy Result To Clipboard.vi"("No. Of Decimal Places (6)"=u32 1, "Input"=w355) -> ()
        }
        frame Enabled {
        }
      }
      n233 = call-poly <vilib>:"1D String Array to Delimited String.vi"("delimiter"="\r\n", "string array"=w330) -> ("delimited string"=w327:string)  [unwired: 9 in]
      "No. Of Iterations As Block Of Text (easy to copy into Excel)" <- w327
      n234 = invoke class="Application" method="Clipboard.Write"("Param 0"=w327) -> (error out=w328:errorcluster)  [unwired: 3 in, 3 out]
      n235 = call <vilib>:"Clear Errors.vi"("error in (no error)"=w328) -> ()  [unwired: 5 in, 2 out]
      "No. Of Iterations Executed - Loop 1" <- w351
      "Output - Loop 1" <- w353
      "No. Of Iterations Executed - Loop 2" <- w350
      "Output - Loop 2" <- w352
      "No. Of Iterations Executed - Loop 3" <- w346
      "Output - Loop 3" <- w348
      "No. Of Iterations Executed - Loop 4" <- w345
      "Output - Loop 4" <- w347
      "No. Of Iterations Executed - Loop 5" <- w337
      "Output - Loop 5" <- w343
      "No. Of Iterations Executed - Loop 6" <- w336
      "Output - Loop 6" <- w342
      "No. Of Iterations Executed - Loop 7" <- w335
      "Output - Loop 7" <- w341
      "No. Of Iterations Executed - Loop 8" <- w334
      "Output - Loop 8" <- w340
      "No. Of Iterations Executed - Loop 9" <- w333
      "Output - Loop 9" <- w339
      "No. Of Iterations Executed - Loop 10" <- w332
      "Output - Loop 10" <- w338
      "No. Of Iterations Executed - Loop 11" <- w325
      "Output - Loop 11" <- w326
    }
  }
